vi "Change Internal-External.vi"() -> ()   [LabVIEW 2019, in "Controller.lvlib"]
uses:
  Controller.lvlib
  Controller Message.ctl
  MDS Command.ctl
  Serial Info.ctl
  UI/Update Message.ctl
  UI/Update Command.ctl
  IMode.ctl
  UI/UI.lvlib
panel:
  out "error out":errorcluster
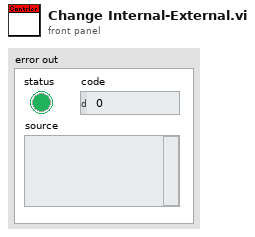
[diagram p1: front panel]
types:
  T1 = typedef "Controller.lvlib/IMode.ctl" = enum8{"Internal", "External"}
  T2 = typedef "UI.lvlib/Update Message.ctl" = cluster{"Update Command":T3, "Channel":u8, "Value":variant}
  T3 = typedef "UI.lvlib/Update Command.ctl" = enum16{"Update Frequency", "Update Power", "Update Switch", "Error", "Stop"}
  T4 = typedef "Controller.lvlib/Serial Info.ctl" = cluster{"Port":refnum<visa-resource-name>, "Baud Rate":u32}
  T5 = typedef "Controller.lvlib/Controller Message.ctl" = cluster{"MDS Command":T6, "Channel":u8, "Value":variant}
  T6 = typedef "Controller.lvlib/MDS Command.ctl" = enum16{"Idle", "Open", "Set VMode", "Set IMode", "Get Frequency", "Set Frequency", "Get Power", "Set Power (dBm)", "Set Power (%)", "Get Switch", "Switch Channel", "Store", "Wait for Prompt", "Wait for State", "Reset", "Error", "Close", "Stop"}
  T7 = typedef "Controller.lvlib/Controller Message Queue.ctl" = refnum<queue>
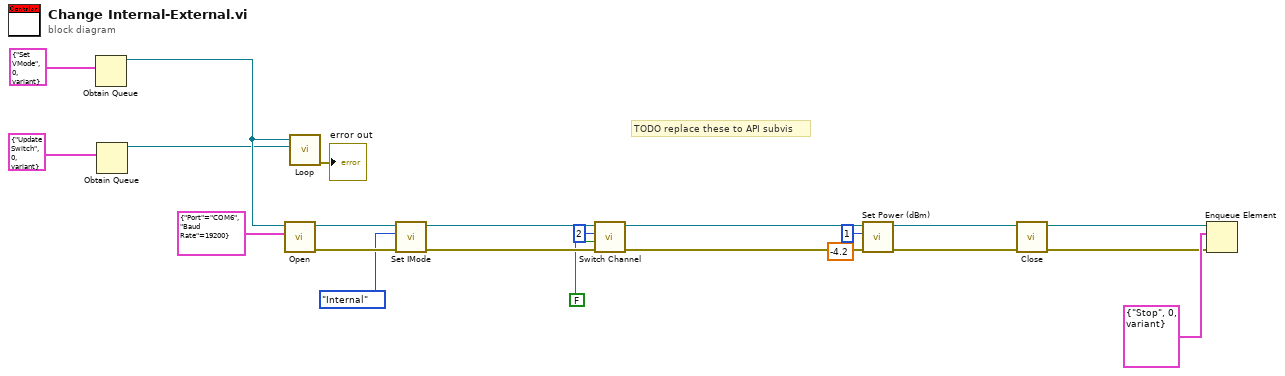
[diagram p0: block diagram]
diagram:
  # "TODO replace these to API subvis"
  n1 = Obtain Queue(element data type=T5 {"MDS Command"=enum."Set VMode", "Channel"=0, "Value"=variant} ("Controller Message")) -> (queue out=w17:refnum<queue>)  [unwired: 4 in, 2 out]
  n2 = Obtain Queue(element data type=T2 {"Update Command"=enum."Update Switch", "Channel"=0, "Value"=variant} ("Controller Message")) -> (queue out=w13:refnum<queue>)  [unwired: 4 in, 2 out]
  n3 = call "Open.vi"("Serial Info"=T4 {"Port"="COM6", "Baud Rate"=19200}, "Controller Queue in"=w17) -> ("error out"=w12:errorcluster, "Controller Queue out"=w16:T7)  [unwired: 8 in]
  n4 = call "Loop.vi"("UI Queue"=w13, "Controller Queue"=w17) -> ("error out"=→"error out":errorcluster)  [unwired: 9 in]
  n5 = call "Set IMode.vi"("error in (no error)"=w12, "IMode (Internal)"=IMode."Internal" ("IMode"), "Queue in"=w16) -> ("error out"=w11:errorcluster, "Queue out"=w20:T7)  [unwired: 7 in]
  n6 = call "Switch Channel.vi"("error in (no error)"=w11, "On/Off"=FALSE, "Channel"=u8 2, "Queue in"=w20) -> ("error out"=w10:errorcluster, "Queue out"=w18:T7)  [unwired: 6 in]
  n7 = call "Set Power (dBm).vi"("error in (no error)"=w10, "Power (dBm)"=-4.2, "Channel"=u8 1, "Queue in"=w18) -> ("error out"=w5:errorcluster, "Queue out"=w6:T7)  [unwired: 6 in]
  n8 = call "Close.vi"("error in (no error)"=w5, "Controller Queue in"=w6) -> ("error out"=w3:errorcluster, "Controller Queue out"=w4:T7)  [unwired: 8 in]
  n9 = Enqueue Element(queue=w4, element=T5 {"MDS Command"=enum."Stop", "Channel"=0, "Value"=variant} ("Controller Message"), error in (no error)=w3) -> ()  [unwired: 1 in, 3 out]
